vi "demo.vi"   [LabVIEW 2010]
uses:
  <vilib>/NXT/Dual Mode Library/Display/drawNumber.vi
types:
  T1 = typedef "LVHSConnector.ctl" = cluster{"Hardware":string, "Flattened String":string}
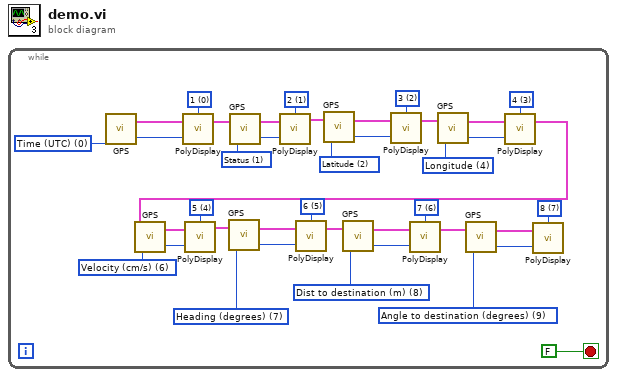
[diagram p0: block diagram]
diagram:
  n1 = while {
    stop <- FALSE stop-if-true
    w1 = i16 7 items=["1", "2", "3", "4", "5", "6", "7", "8"] ("Line")
    w4 = u16 9 items=["Time (UTC)"=0, "Status"=1, "Latitude"=2, "Longitude"=4, "Velocity (cm/s)"=6, "Heading (degrees)"=7, "Dist to destination (m)"=8, "Angle to destination (degrees)"=9, "Angle since last req"=10, "Set Destination Latitude"=11, "Set Destination Longitude"=12] ("Data Requested")
    w19 = i16 6 items=["1", "2", "3", "4", "5", "6", "7", "8"] ("Line")
    w20 = u16 8 items=["Time (UTC)"=0, "Status"=1, "Latitude"=2, "Longitude"=4, "Velocity (cm/s)"=6, "Heading (degrees)"=7, "Dist to destination (m)"=8, "Angle to destination (degrees)"=9, "Angle since last req"=10, "Set Destination Latitude"=11, "Set Destination Longitude"=12] ("Data Requested")
    w14 = i16 5 items=["1", "2", "3", "4", "5", "6", "7", "8"] ("Line")
    w10 = i16 4 items=["1", "2", "3", "4", "5", "6", "7", "8"] ("Line")
    w9 = u16 7 items=["Time (UTC)"=0, "Status"=1, "Latitude"=2, "Longitude"=4, "Velocity (cm/s)"=6, "Heading (degrees)"=7, "Dist to destination (m)"=8, "Angle to destination (degrees)"=9, "Angle since last req"=10, "Set Destination Latitude"=11, "Set Destination Longitude"=12] ("Data Requested")
    w3 = u16 6 items=["Time (UTC)"=0, "Status"=1, "Latitude"=2, "Longitude"=4, "Velocity (cm/s)"=6, "Heading (degrees)"=7, "Dist to destination (m)"=8, "Angle to destination (degrees)"=9, "Angle since last req"=10, "Set Destination Latitude"=11, "Set Destination Longitude"=12] ("Data Requested")
    w24 = i16 3 items=["1", "2", "3", "4", "5", "6", "7", "8"] ("Line")
    w23 = u16 4 items=["Time (UTC)"=0, "Status"=1, "Latitude"=2, "Longitude"=4, "Velocity (cm/s)"=6, "Heading (degrees)"=7, "Dist to destination (m)"=8, "Angle to destination (degrees)"=9, "Angle since last req"=10, "Set Destination Latitude"=11, "Set Destination Longitude"=12] ("Data Requested")
    w29 = i16 2 items=["1", "2", "3", "4", "5", "6", "7", "8"] ("Line")
    w33 = i16 1 items=["1", "2", "3", "4", "5", "6", "7", "8"] ("Line")
    w34 = i16 0 items=["1", "2", "3", "4", "5", "6", "7", "8"] ("Line")
    w37 = u16 2 items=["Time (UTC)"=0, "Status"=1, "Latitude"=2, "Longitude"=4, "Velocity (cm/s)"=6, "Heading (degrees)"=7, "Dist to destination (m)"=8, "Angle to destination (degrees)"=9, "Angle since last req"=10, "Set Destination Latitude"=11, "Set Destination Longitude"=12] ("Data Requested")
    w38 = u16 1 items=["Time (UTC)"=0, "Status"=1, "Latitude"=2, "Longitude"=4, "Velocity (cm/s)"=6, "Heading (degrees)"=7, "Dist to destination (m)"=8, "Angle to destination (degrees)"=9, "Angle since last req"=10, "Set Destination Latitude"=11, "Set Destination Longitude"=12] ("Data Requested")
    w40 = u16 0 items=["Time (UTC)"=0, "Status"=1, "Latitude"=2, "Longitude"=4, "Velocity (cm/s)"=6, "Heading (degrees)"=7, "Dist to destination (m)"=8, "Angle to destination (degrees)"=9, "Angle since last req"=10, "Set Destination Latitude"=11, "Set Destination Longitude"=12] ("Data Requested")
    n2 = call "GPS.vi"("Data Requested"=w40) -> ("value"=w35:i32, "NXT"=w39:T1)  [unwired: 2 in]
    n3 = call-poly <vilib>:"PolyDisplay.vi"("number"=w35, "NXT"=w39, "Line"=w34) -> ("NXT"=w36:T1)  [unwired: 1 in]
    n4 = call "GPS.vi"("Data Requested"=w38, "NXT"=w36) -> ("value"=w32:i32, "NXT"=w31:T1)  [unwired: 1 in]
    n5 = call-poly <vilib>:"PolyDisplay.vi"("number"=w32, "NXT"=w31, "Line"=w33) -> ("NXT"=w30:T1)  [unwired: 1 in]
    n6 = call "GPS.vi"("Data Requested"=w37, "NXT"=w30) -> ("value"=w28:i32, "NXT"=w27:T1)  [unwired: 1 in]
    n7 = call-poly <vilib>:"PolyDisplay.vi"("number"=w28, "NXT"=w27, "Line"=w29) -> ("NXT"=w22:T1)  [unwired: 1 in]
    n8 = call "GPS.vi"("Data Requested"=w23, "NXT"=w22) -> ("value"=w25:i32, "NXT"=w26:T1)  [unwired: 1 in]
    n9 = call-poly <vilib>:"PolyDisplay.vi"("number"=w25, "NXT"=w26, "Line"=w24) -> ("NXT"=w8:T1)  [unwired: 1 in]
    n10 = call "GPS.vi"("Data Requested"=w3, "NXT"=w8) -> ("value"=w11:i32, "NXT"=w12:T1)  [unwired: 1 in]
    n11 = call-poly <vilib>:"PolyDisplay.vi"("number"=w11, "NXT"=w12, "Line"=w10) -> ("NXT"=w13:T1)  [unwired: 1 in]
    n12 = call "GPS.vi"("Data Requested"=w9, "NXT"=w13) -> ("value"=w15:i32, "NXT"=w16:T1)  [unwired: 1 in]
    n13 = call-poly <vilib>:"PolyDisplay.vi"("number"=w15, "NXT"=w16, "Line"=w14) -> ("NXT"=w21:T1)  [unwired: 1 in]
    n14 = call "GPS.vi"("Data Requested"=w20, "NXT"=w21) -> ("value"=w18:i32, "NXT"=w17:T1)  [unwired: 1 in]
    n15 = call-poly <vilib>:"PolyDisplay.vi"("number"=w18, "NXT"=w17, "Line"=w19) -> ("NXT"=w5:T1)  [unwired: 1 in]
    n16 = call "GPS.vi"("Data Requested"=w4, "NXT"=w5) -> ("value"=w6:i32, "NXT"=w7:T1)  [unwired: 1 in]
    n17 = call-poly <vilib>:"PolyDisplay.vi"("number"=w6, "NXT"=w7, "Line"=w1) -> ()  [unwired: 1 in, 1 out]
  }
